vi "MISSION_CLEAR_ALL.vi"(0 "target_system":u8=6, 5 "target_component":u8=8) -> (4 "MAVLink Message":u8[](array[numeric]))   [LabVIEW 2014]
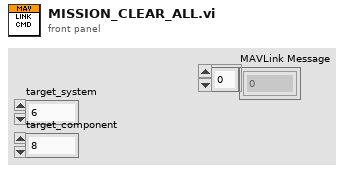
[diagram p1: front panel]
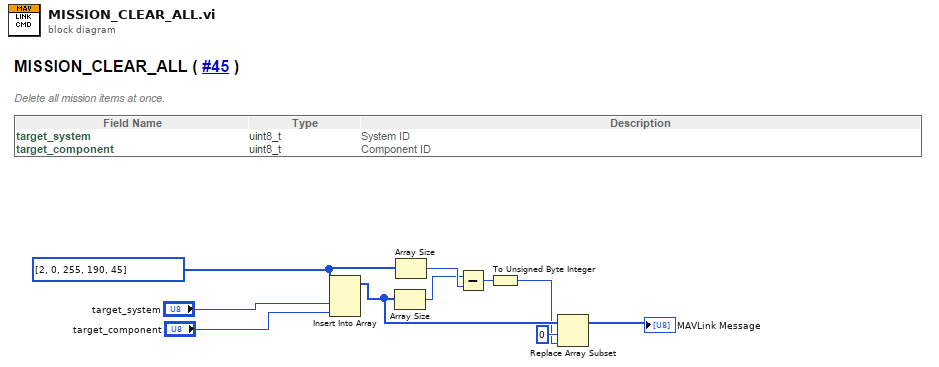
[diagram p0: block diagram]
diagram:
  w10 = u8[] [2, 0, 255, 190, 45]
  n1 = Insert Into Array(array=w10, new element #1="target_system", new element #2="target_component") -> (w6:u8[])  [unwired: 1 in]
  n2 = Array Size(array=w6) -> (size(s)=w8:i32)
  n3 = Array Size(array=w10) -> (size(s)=w9:i32)
  n4 = Subtract(x=w8, y=w9) -> (x-y=w7:i32)
  n5 = To Unsigned Byte Integer(number=w7) -> (unsigned 8bit integer=w4:u8)
  n6 = Replace Array Subset(array=w6, new element=w4, index=0) -> (→"MAVLink Message":u8[])
